vi "get-video-ROIs.vi"() -> ()   [LabVIEW 2024]
uses:
  <vilib>/vision/NI_Vision_Development_Module.lvlib
panel:
  out "Codec Names":string[](array[string])
  in  "GRABAR":bool
  in  "stop":bool
  out "Full Image":T1(plugin-control)
  out "error out":errorcluster
  out "Ojo":T1(plugin-control)
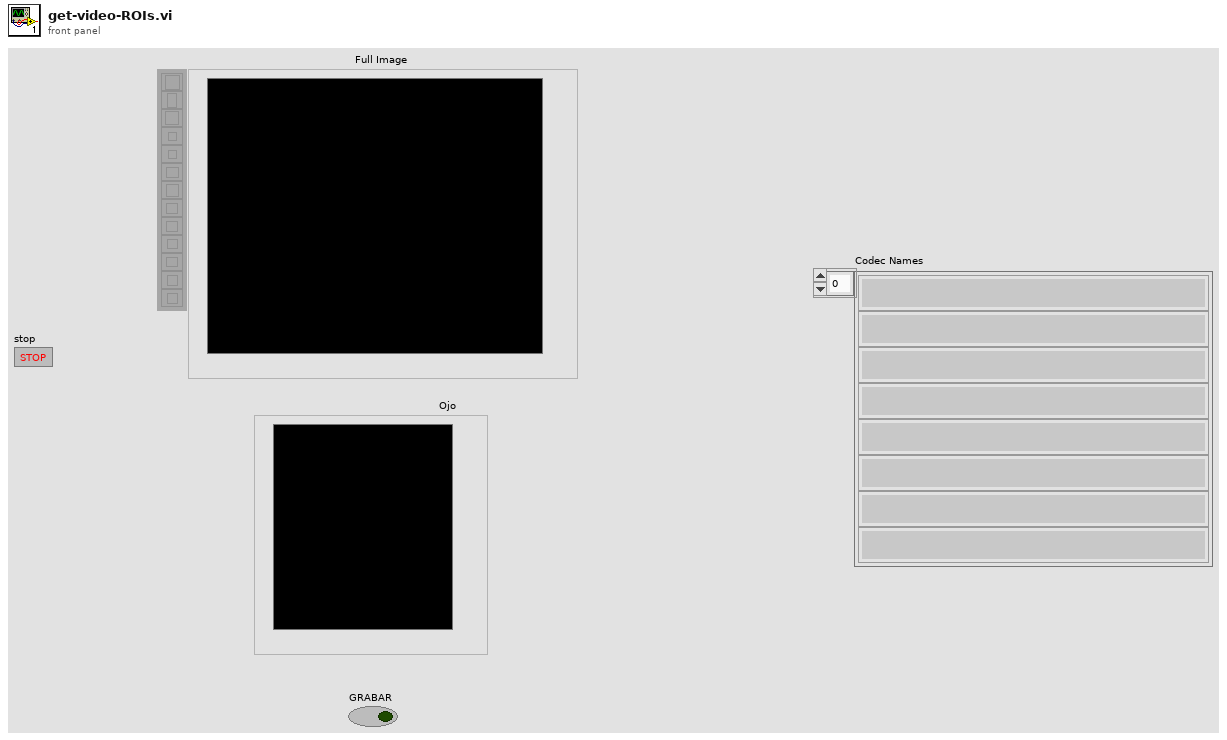
[diagram p1: front panel]
types:
  T1 = typedef "IMAQ Image.ctl" = refnum<image>
  T2 = typedef "Image Type" = u32
  T3 = typedef "IMAQ AVI2 Refnum.ctl" = refnum<k20>
  T4 = cluster{"Global Rectangle":i32[], "Contours":cluster{"Contour Type":u32, "ROI Type":u32, "Points":i32[]}[]}
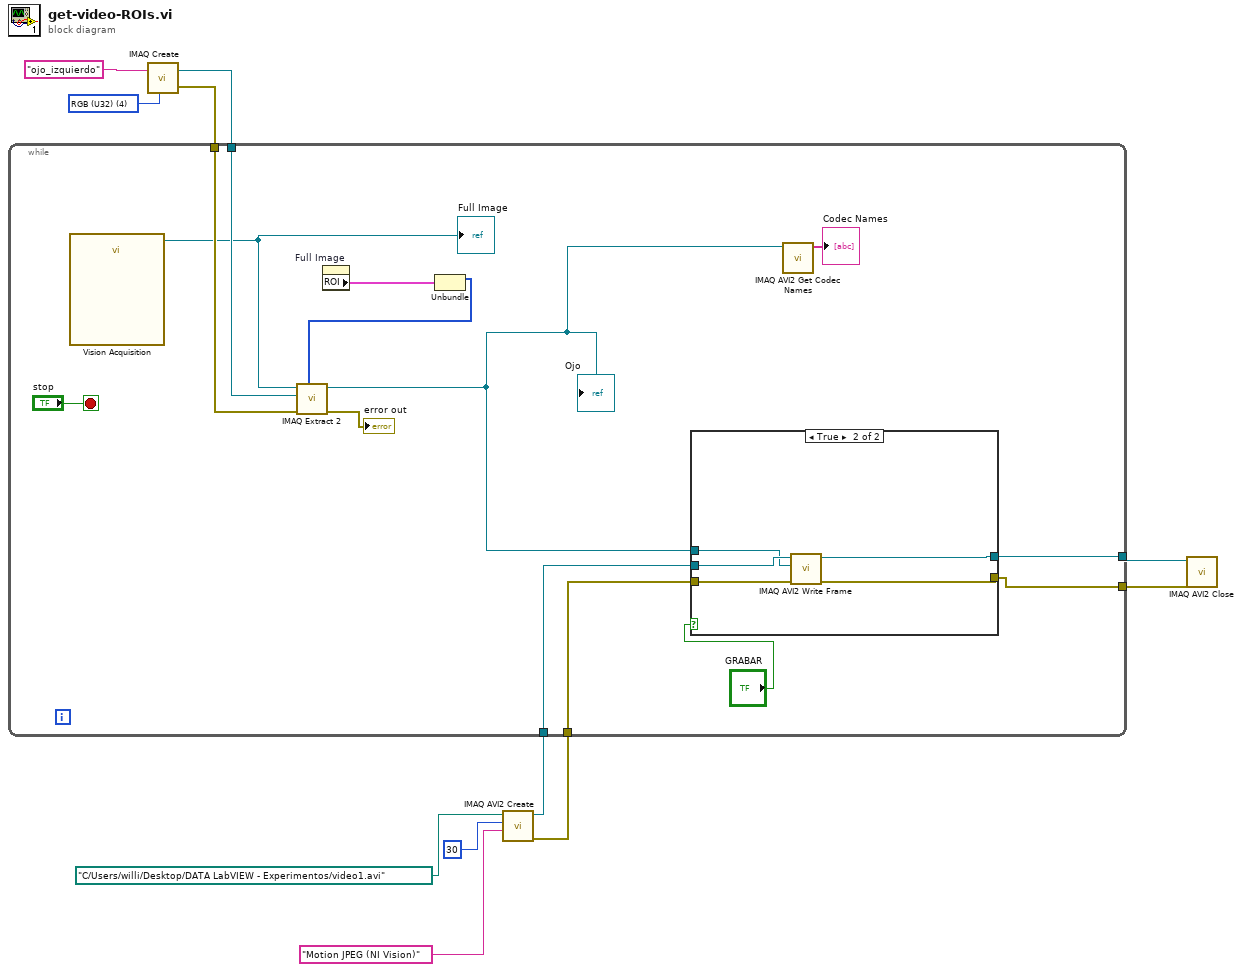
[diagram p0: block diagram]
diagram:
  w10 = T2 4 items=["Grayscale (U8)", "Grayscale (I16)", "Grayscale (SGL)", "Complex (CSG)", "RGB (U32)", "HSL (U32)", "RGB (U64)", "Grayscale (U16)"] ("Image Type")
  n1 = call "IMAQ Create"("Image Name"="ojo_izquierdo", "Image Type"=w10) -> ("New Image"=w8:T1, "error out"=w9:errorcluster)  [unwired: 3 in]
  n2 = call "IMAQ AVI2 Create"("Codec"="Motion JPEG (NI Vision)", "Frames Per Second"=u32 30, "AVI Path"=path "C:/Users/willi/Desktop/DATA LabVIEW - Experimentos/video1.avi") -> ("error out"=w4:errorcluster, "AVI Refnum"=w3:T3)  [unwired: 7 in]
  n3 = while {
    tunnel: w9 -> [w24]
    tunnel: w8 -> [w23]
    tunnel: w4 -> [w15]
    tunnel: w3 -> [w14]
    tunnel: [w13] -> w2
    tunnel: [w12] -> w1
    stop <- "stop" stop-if-true
    n4 = call "Vision Acquisition"() -> ("Image Out"=w19:T1)  [unwired: 25 in, 2 out]
    "Full Image" <- w19
    n5 = property on="Full Image" class="ImageControl"() -> ("ROI"=w22:T4)  [unwired: 2 in, 2 out]
    n6 = Unbundle "Unbundle"(w22) -> ("Global Rectangle"=w21:i32[])  [unwired: 1 out]
    n7 = call "IMAQ Extract 2"("Optional Rectangle"=w21, "error in (no error)"=w24, "Image Dst"=w23, "Image Src"=w19) -> ("error out"=→"error out":errorcluster, "Image Dst Out"=w17:T1)  [unwired: 6 in]
    "Ojo" <- w17
    n8 = case shown="True" "GRABAR" {
      tunnel: w14 -> [w27 w32]
      tunnel: w15 -> [w26 w31]
      tunnel: [w26 w30] -> w13
      tunnel: [w27 w29] -> w12
      tunnel: w17 -> [_ w28]
      frame False {
      }
      frame True {
        n9 = call "IMAQ AVI2 Write Frame"("error in (no error)"=w31, "Image"=w28, "AVI Refnum"=w32) -> ("error out"=w30:errorcluster, "AVI Refnum (duplicate)"=w29:T3)  [unwired: 6 in, 1 out]
      }
    }
    n10 = call "IMAQ AVI2 Get Codec Names"("Image"=w17) -> ("Codec Names"=→"Codec Names":string[])  [unwired: 9 in, 1 out]
  }
  n11 = call "IMAQ AVI2 Close"("error in (no error)"=w2, "AVI Refnum"=w1) -> ()  [unwired: 9 in, 1 out]
